vi "Prompt Retrieve Key Array for Config.vi"(8 "error in (no error)":errorcluster, 10 "Key Array In":T3, 11 "Connection Refnum":T1) -> (0 "error out":errorcluster, 2 "Prompt Test Parameters":T2, 3 "Connection Refnum":T1)   [LabVIEW 2011]
uses:
  ITK/utils/keyedarr.llb/Keyed Array.ctl
  TypeDefs/Prompt Test Parameters.ctl
  Summitek/Win32/ODBC/SQL Controls/Connection Refnum.ctl
  ITK/utils/strutil.llb/Case Matching.ctl
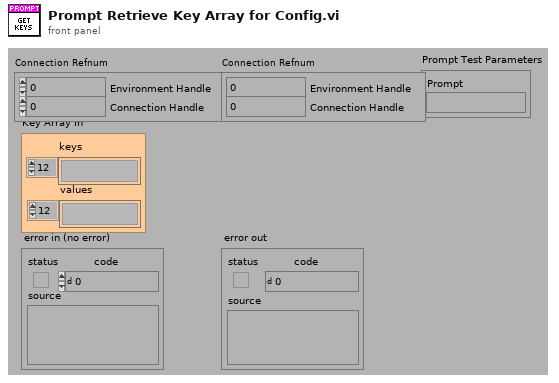
[diagram p1: front panel]
types:
  T1 = typedef "Connection Refnum.ctl" = cluster{"Environment Handle":i32, "Connection Handle":i32}
  T2 = typedef "Prompt Test Parameters.ctl" = cluster{"Prompt":string}
  T3 = typedef "Keyed Array.ctl" = cluster{"keys":string[], "values":string[]}
  T4 = typedef "Case Matching.ctl" = enum16{"a != A", "a == A", "system"}
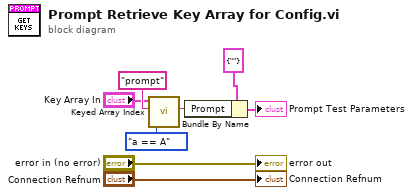
[diagram p0: block diagram]
diagram:
  n1 = call "Keyed Array Index.vi"("case matching (sensitive)"=Case_Matching."a == A", "key"="prompt", "array in"="Key Array In") -> ("value"=w1:string)  [unwired: 1 in, 3 out]
  n2 = Bundle By Name(cluster=T2 {"Prompt"=""} ("Prompt Test Parameters"), "Prompt"=w1) -> (→"Prompt Test Parameters":T2)
  "error out" <- "error in (no error)"
  "Connection Refnum" <- "Connection Refnum"
